vi "Launch Actor.vi"() -> ()   [LabVIEW 2018, in "Counter.lvclass"]
uses:
  Counter Class/Counter.lvclass
  Message Class/Message.lvclass
panel:
  out "Self Queue":refnum<queue>
  out "error out":errorcluster
  in  "Queue for message Queue":refnum<queue>
  in  "Caller_Queue":refnum<queue>
  in  "Counter.lvclass":refnum<class "Counter.lvclass">
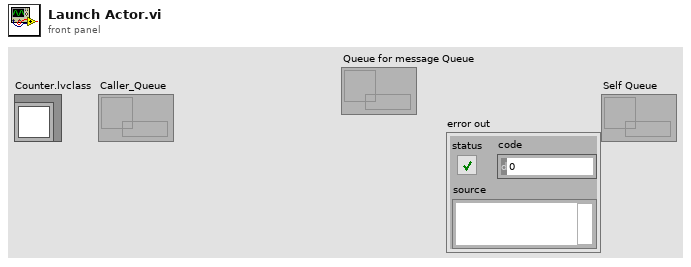
[diagram p1: front panel]
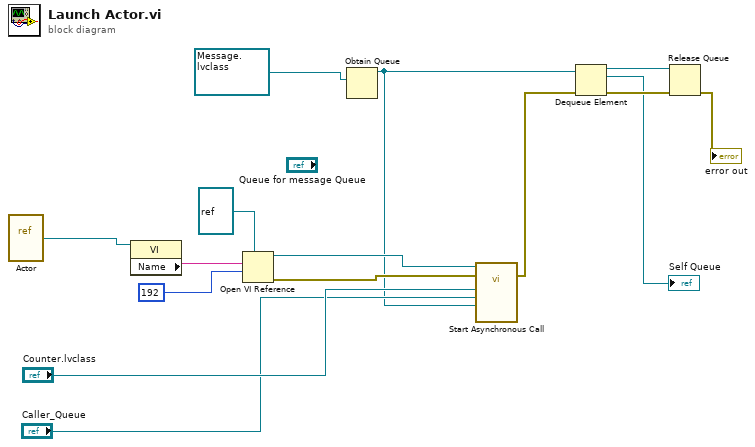
[diagram p0: block diagram]
diagram:
  n1 = vi-ref "Actor.vi"() -> (w12:refnum<vi>)
  n2 = property class="VI"(reference=w12) -> ("Name"=w13:string)  [unwired: 1 in, 2 out]
  n3 = Open VI Reference(type specifier VI Refnum (for type only)=refnum<vi> refnum, vi path=w13, options=192) -> (vi reference=w10:refnum<vi>, error out=w14:errorcluster)  [unwired: 3 in]
  n4 = Obtain Queue(element data type=refnum<queue> refnum ("queue out")) -> (queue out=w6:refnum<queue>)  [unwired: 4 in, 2 out]
  n5 = call-by-ref "Start Asynchronous Call"(reference=w10, error in=w14, "Queue for message Queue"=w6, "Caller_Queue"="Caller_Queue", "Actor Input"="Counter.lvclass") -> (error out=w5:errorcluster)  [unwired: 8 in, 2 out]
  n6 = Dequeue Element(queue=w6, error in (no error)=w5) -> (queue out=w4:refnum<queue>, element=→"Self Queue":refnum<queue>, error out=w3:errorcluster)  [unwired: 1 in, 1 out]
  n7 = Release Queue(queue=w4, error in (no error)=w3) -> (error out=→"error out":errorcluster)  [unwired: 1 in, 2 out]
